vi "ni5660 Sub Set Multi-Span Settings.vi"(0 "receiver info in":T2, 5 "multispan settings":T1 {"df" format="%.2f"; "fc adjustment" format="%.2f"; "segment size" format="%.2f"; "frequency shifts" format="%.2f"}, 11 "error in (no error)":errorcluster) -> (4 "receiver info out":T2, 15 "error out":errorcluster)   [LabVIEW 2011]
uses:
  <vilib>/addons/Modulation/niScope/controls/mod_Modulation Settings.ctl
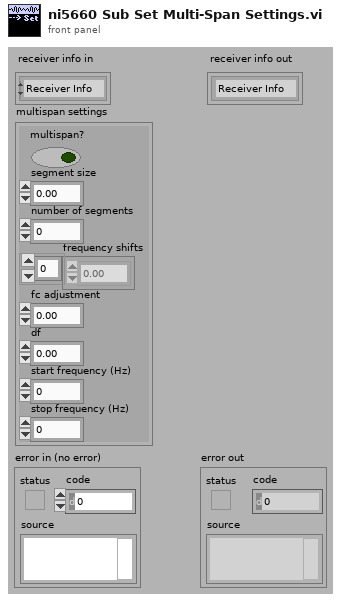
[diagram p1: front panel]
types:
  T1 = cluster{"multispan?":bool, "segment size":dbl, "number of segments":i32, "frequency shifts":dbl[], "fc adjustment":dbl, "df":dbl, "start frequency (Hz)":dbl, "stop frequency (Hz)":dbl}
  T2 = typedef "mod_Modulation Settings.ctl" = cluster{enum16{"Receiver Info"}, variant}
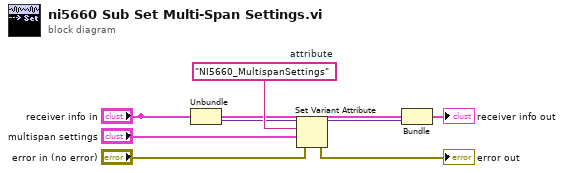
[diagram p0: block diagram]
diagram:
  w8 = "NI5660_MultispanSettings"  # attribute
  n1 = Unbundle("receiver info in") -> (w4:variant)  [unwired: 1 out]
  n2 = Set Variant Attribute(Variant=w4, name=w8, value="multispan settings", error in="error in (no error)") -> (Variant out=w3:variant, error out=→"error out":errorcluster)  [unwired: 1 out]
  n3 = Bundle(cluster="receiver info in", w3) -> (→"receiver info out":T2)  [unwired: 1 in]
